vi "Start Recipe.vi"(8 "error in (no error)":errorcluster, 10 "Recipe File":path, 11 "Recipe Process in":refnum<class "Recipe Process.lvclass">) -> (0 "error out":errorcluster, 3 "Recipe Process out":refnum<class "Recipe Process.lvclass">)   [LabVIEW 2022 SP3, in "Recipe Process.lvlib" / "Recipe Process.lvclass"]
uses:
  Recipe Process.lvclass
  Single Recipe Step.ctl
  Recipe XY Position.ctl
  Recipe Process.lvclass/Recipe Process.ctl
  XY Stage/Process Actor/Process Framework/Process State Data/Process State Data.lvclass/Process State Data.ctl
  Recipe State Data/Recipe State Data.lvclass/Recipe State Data.ctl
  XY Stage/Process Actor/Process Framework/Process State Data/Accessor/Read Abort.vi
  Recipe State Data/Write Current Recipe Iterations.vi
  Recipe State Data/Write Desired Recipe Iterations.vi
  XY Stage/Process Actor/Process Framework/Process State Data/Process State Data.lvclass
  Recipe State Data/Recipe State Data.lvclass
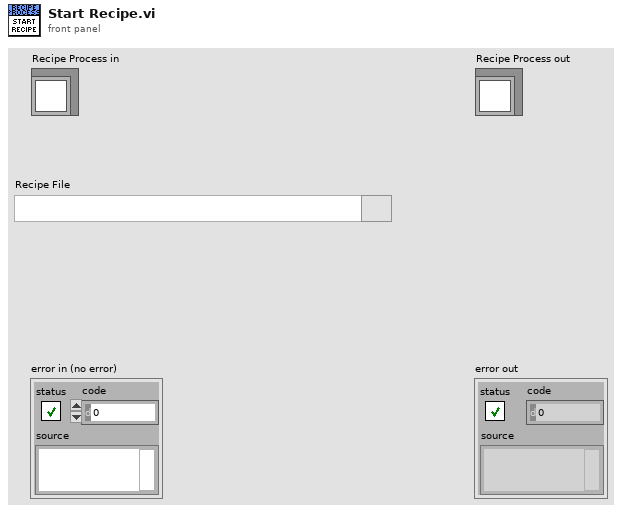
[diagram p1: front panel]
types:
  T1 = typedef "Recipe Process.lvlib/Recipe Process.lvclass/Single Recipe Step.ctl" = cluster{"XY Position":T2, "Laser Power":dbl, "AI Aquisition Time(s)":dbl}
  T2 = typedef "Recipe Process.lvlib/Recipe Process.lvclass/Recipe XY Position.ctl" = cluster{"X Position":dbl, "Y Position":dbl}
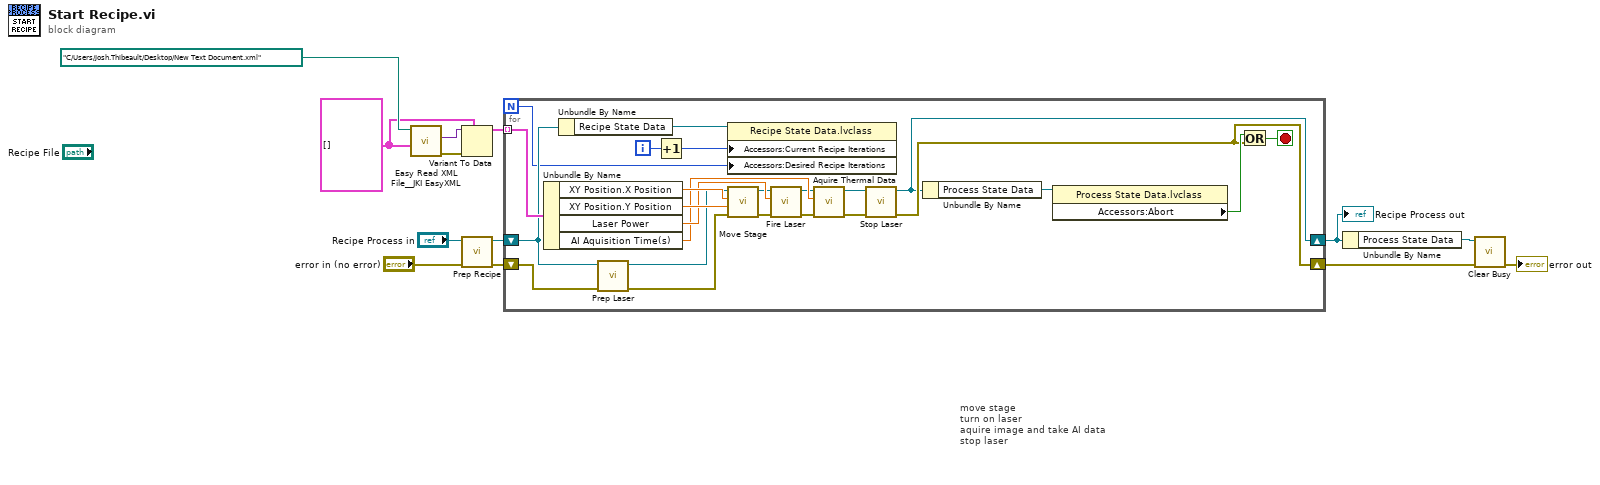
[diagram p0: block diagram]
diagram:
  w1 = T1[] [] ("Array")
  # "move stage\nturn on laser\naquire image and take AI data\nstop laser"
  n1 = call <vilib>:"Easy Read XML File__JKI EasyXML.vi"("LabVIEW Data (Type)"=w1, "XML File Path"=path "C:/Users/Josh.Thibeault/Desktop/New Text Document.xml") -> ("error out"=w9:errorcluster, "LabVIEW Data"=w8:variant)  [unwired: 7 in, 1 out]
  n2 = Variant To Data(error in=w9, type=w1, Variant=w8) -> (data=w7:T1[])  [unwired: 1 out]
  n3 = call "Prep Recipe.vi"("error in (no error)"="error in (no error)", "Recipe Process in"="Recipe Process in") -> ("error out"=w10:errorcluster, "Recipe Process out"=w11:refnum<class "Recipe Process.lvclass">)  [unwired: 8 in]
  n4 = for {
    N -> [w15]
    shift-right: [w22] -> w6
    shift-left: w11 -> [w18]
    shift-right: [w24] -> w4
    shift-left: w10 -> [w20]
    tunnel: w7 -> [w37] mode=indexing
    i -> [w16]
    stop <- w27 stop-if-true
    n5 = Unbundle By Name(w37) -> ("XY Position.X Position"=w36:dbl, "XY Position.Y Position"=w35:dbl, "Laser Power"=w34:dbl, "AI Aquisition Time(s)"=w31:dbl)
    n6 = Unbundle By Name(w18) -> ("Recipe State Data"=w17:refnum<data-value>)
    n7 = call "Prep Laser.vi"("error in (no error)"=w20, "Recipe Process in"=w18) -> ("error out"=w19:errorcluster, "Recipe Process"=w21:refnum<class "Recipe Process.lvclass">)  [unwired: 8 in]
    n8 = Increment(x=w16) -> (x+1=w14:i32)
    n9 = property class="Recipe State Data.lvclass"(reference=w17, "Accessors:Current Recipe Iterations"=w14, "Accessors:Desired Recipe Iterations"=w15) -> ()  [unwired: 1 in, 2 out]
    n10 = call "Move Stage.vi"("error in (no error)"=w19, "Y Position"=w35, "X Position"=w36, "Recipe Process in"=w21) -> ("error out"=w33:errorcluster, "Recipe Process out"=w32:refnum<class "Recipe Process.lvclass">)  [unwired: 6 in]
    n11 = call "Fire Laser.vi"("error in (no error)"=w33, "Laser Power"=w34, "Recipe Process in"=w32) -> ("error out"=w30:errorcluster, "Recipe Process out"=w29:refnum<class "Recipe Process.lvclass">)  [unwired: 7 in]
    n12 = call "Aquire Thermal Data.vi"("error in (no error)"=w30, "AI Aquisition Time(s)"=w31, "Recipe Process in"=w29) -> ("error out"=w25:errorcluster, "Recipe Process out"=w23:refnum<class "Recipe Process.lvclass">)  [unwired: 7 in]
    n13 = call "Stop Laser.vi"("error in (no error)"=w25, "Recipe Process in"=w23) -> ("error out"=w24:errorcluster, "Recipe Process out"=w22:refnum<class "Recipe Process.lvclass">)  [unwired: 8 in]
    n14 = Unbundle By Name(w22) -> ("Process State Data"=w26:refnum<data-value>)
    n15 = property class="Process State Data.lvclass"(reference=w26) -> ("Accessors:Abort"=w28:bool)  [unwired: 1 in, 2 out]
    n16 = Or(x=w28, y=w24) -> (x .or. y?=w27:bool)
  }
  "Recipe Process out" <- w6
  n17 = Unbundle By Name(w6) -> ("Process State Data"=w5:refnum<data-value>)
  n18 = call "Clear Busy.vi"("error in (no error)"=w4, "Process State"=w5) -> ("error out"=→"error out":errorcluster)  [unwired: 8 in, 1 out]
